vi "Create.vi"(8 "error in (no error)":errorcluster, 11 "Configuration":path) -> (0 "error out":errorcluster, 3 "Room-API out":refnum<class "Room-API.lvclass">)   [LabVIEW 2020, in "Room-API.lvclass"]
uses:
  Room-API.lvclass
  Room-API.lvclass/Room-API.ctl
  <vilib>/ErrorRing/Error Ring.xnode
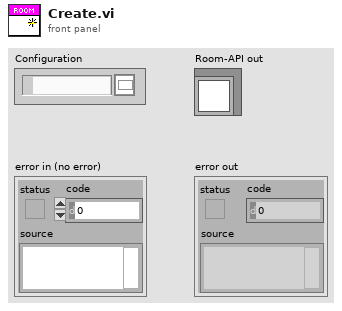
[diagram p1: front panel]
types:
  T1 = typedef "Room-API.lvclass/Single Room.ctl" = cluster{"name":string, "temperature_humidity":string[], "bond":string[], "hue":string[]}
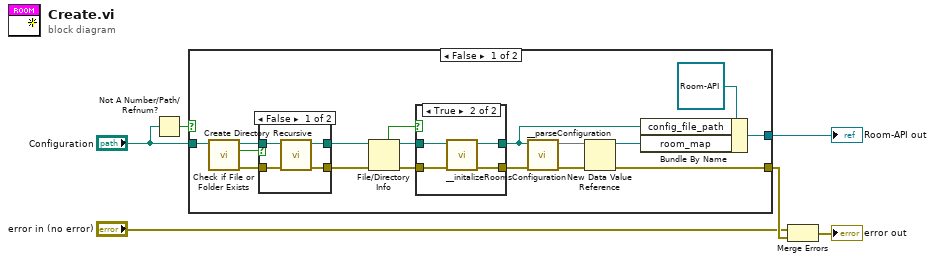
[diagram p0: block diagram]
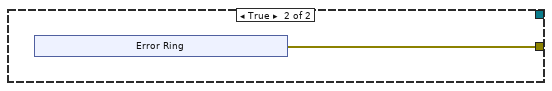
[diagram p4: hidden frame]
diagram:
  n1 = Not A Number/Path/Refnum?(number/path/refnum="Configuration") -> (NaN/Path/Refnum?=w6:bool)
  n2 = case shown="False" w6 {
    tunnel: "Configuration" -> [w23 _]
    tunnel: [w11 w36] -> w3
    tunnel: [w8 _] -> w4
    frame False {
      n3 = call <vilib>:"Check if File or Folder Exists.vi"("path"=w23) -> ("error out"=w20:errorcluster, "file or folder exists?"=w22:bool, "dup path"=w21:path)  [unwired: 8 in]
      n4 = case shown="False" w22 {
        tunnel: w21 -> [w33 w35]
        tunnel: w20 -> [w31 w34]
        tunnel: [w32 w35] -> w15
        tunnel: [w30 w34] -> w14
        frame False {
          n5 = call <vilib>:"Create Directory Recursive.vi"("error in (no error)"=w31, "directory"=w33) -> ("error out"=w30:errorcluster, "directory copy"=w32:path)  [unwired: 3 in, 1 out]
        }
        frame True {
        }
      }
      n6 = File/Directory Info(path=w15, error in=w14) -> (path out=w18:path, directory=w19:bool, error out=w17:errorcluster)  [unwired: 4 out]
      n7 = case shown="True" w19 {
        tunnel: w18 -> [w24 w29]
        tunnel: [w24 w28] -> w9
        tunnel: [w25 w27] -> w16
        tunnel: w17 -> [w25 w26]
        frame False {
        }
        frame True {
          n8 = call "__initalizeRoomsConfiguration.vi"("error in"=w26, "path in"=w29) -> ("error out"=w27:errorcluster, "file path out"=w28:path)  [unwired: 8 in]
        }
      }
      n9 = call "__parseConfiguration.vi"("error in"=w16, "configFilePath"=w9) -> ("error out"=w13:errorcluster, "room_map"=w12:map{string, T1})  [unwired: 8 in]
      n10 = New Data Value Reference(data value=w12, error in=w13) -> (data value reference=w7:refnum<data-value>, error out=w11:errorcluster)
      n11 = Bundle By Name(cluster=refnum<class "Room-API.lvclass"> refnum ("Room-API.lvclass"), "config_file_path"=w9, "room_map"=w7) -> (w8:refnum<class "Room-API.lvclass">)
    }
    frame True {
      n12 = xnode "Error Ring"() -> ("error out"=w36:errorcluster)
    }
  }
  "Room-API out" <- w4
  n13 = Merge Errors("error in (no error)", w3) -> (→"error out":errorcluster)
